vi "Get Absolute Source Dir Path.vi"() -> (0 "error out":errorcluster, 3 "source dir":path)   [LabVIEW 2021]
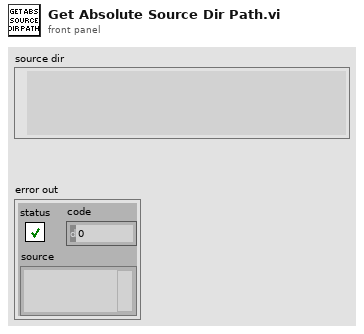
[diagram p1: front panel]
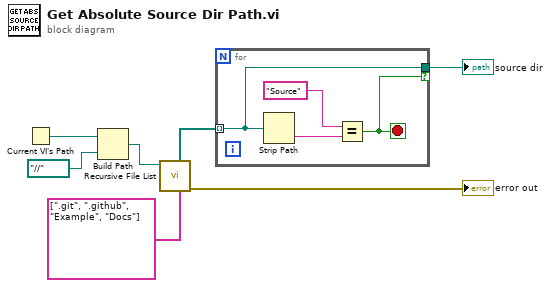
[diagram p0: block diagram]
diagram:
  n1 = Current VI's Path() -> (path=w7:path)
  n2 = Build Path(base path=w7, name or relative path=path "../../..") -> (appended path=w5:path)
  n3 = call <vilib>:"Recursive File List.vi"("Folders to Exclude"=string[] [".git", ".github", "Example", "Docs"], "Folder Path"=w5) -> ("error out"=→"error out":errorcluster, "All Folders"=w1:path[])  [unwired: 5 in, 3 out]
  n4 = for {
    tunnel: w1 -> [w9] mode=indexing
    tunnel: [w9] -> w4 if=w8
    stop <- w8 stop-if-true
    n5 = Strip Path(path=w9) -> (name=w11:string)  [unwired: 1 out]
    n6 = Equal?(x="Source", y=w11) -> (x = y?=w8:bool)
  }
  "source dir" <- w4
